vi "Internal Message Loop.vi"(8 "error in (no error)":errorcluster, 11 "WAMP Client in":refnum<class "WAMP Client.lvclass">) -> (0 "error out":errorcluster, 3 "WAMP Client out":refnum<class "WAMP Client.lvclass">)   [LabVIEW 2020, in "wamplv.lvlib" / "WAMP Client.lvclass"]
uses:
  <userlib>/wamplv/WAMP Client/WAMP Client.lvclass
  <userlib>/wamplv/WAMP Client/TypeDef/SUBSCRIBE Requests Map.ctl
  <userlib>/wamplv/WAMP Client/TypeDef/SUBSCRIBE Request Data.ctl
  <userlib>/wamplv/WAMP Client/TypeDef/Subscribe Result.ctl
  <userlib>/wamplv/WAMP Client/TypeDef/Event Payload.ctl
  <userlib>/wamplv/WAMP Client/TypeDef/Subscriptions Map.ctl
  <userlib>/wamplv/WAMP Client/TypeDef/Subscription Details.ctl
  <userlib>/wamplv/WAMP Client/TypeDef/Unsubscribe Requests Map.ctl
  <userlib>/wamplv/WAMP Client/TypeDef/UNSUBSCRIBE Request Data.ctl
  <userlib>/wamplv/WAMP Client/TypeDef/UNSUBSCRIBE Result.ctl
  <userlib>/wamplv/WAMP Client/TypeDef/Message Loop Shift Reg Data.ctl
  <userlib>/wamplv/WAMP Client/TypeDef/REGISTER Request Data.ctl
  <userlib>/wamplv/WAMP Client/TypeDef/REGISTERED or ERROR payload.ctl
  <userlib>/wamplv/WAMP Client/TypeDef/WAMP Error Payload.ctl
  <userlib>/wamplv/WAMP Client/TypeDef/INVOCATION payload.ctl
  <userlib>/wamplv/WAMP Client/TypeDef/Publish Requests Map.ctl
  <userlib>/wamplv/WAMP Client/TypeDef/PUBLISH Request Data.ctl
  <userlib>/wamplv/WAMP Client/TypeDef/PUBLISH Result.ctl
  <userlib>/wamplv/WAMP Client/TypeDef/Endpoint Data.ctl
  <userlib>/wamplv/WAMP Client/TypeDef/CALL Request Map.ctl
  <userlib>/wamplv/WAMP Client/TypeDef/CALL Request Data.ctl
  <userlib>/wamplv/WAMP Client/TypeDef/RESULT Payload.ctl
  <userlib>/wamplv/WAMP Client/WAMP Client.lvclass/WAMP Client.ctl
  <userlib>/wamplv/WAMP Client/TypeDef/WAMP Received Message.ctl
  <userlib>/wamplv/WAMP Message Codes.ctl
  <userlib>/wamplv/WAMP Client/TypeDef/Termination Reason Enum.ctl
  <userlib>/wamplv/WAMP Client/TypeDef/GOODBYE Request Data.ctl
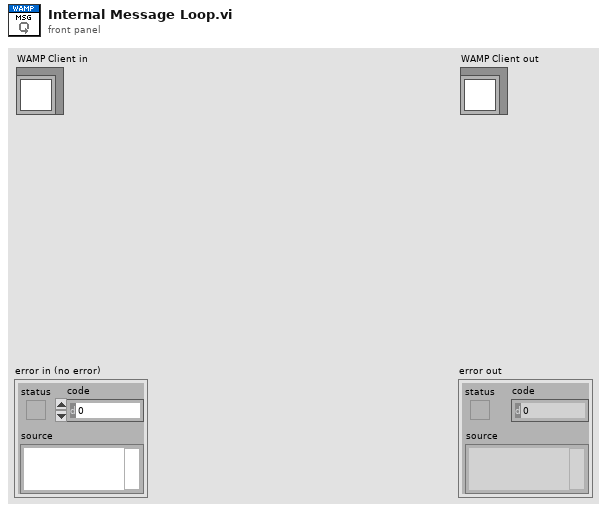
[diagram p1: front panel]
types:
  T1 = typedef "wamplv.lvlib/WAMP Client.lvclass/Message Loop Shift Reg Data.ctl" = cluster{"Register Requests":map{u32, T2}, "Last Request ID":u32, "Publish Requests":T3, "Endpoints Map":map{u32, T5}, "Call Requests":T6}
  T2 = typedef "wamplv.lvlib/WAMP Client.lvclass/REGISTER Request Data.ctl" = cluster{"Procedure URI":string, "Options":string, "REGISTERED or ERROR event":refnum<user-event>, "INVOCATION event":refnum<user-event>}
  T3 = typedef "wamplv.lvlib/WAMP Client.lvclass/Publish Requests Map.ctl" = map{u32, T4}
  T4 = typedef "wamplv.lvlib/WAMP Client.lvclass/PUBLISH Request Data.ctl" = cluster{"Topic URI":string, "Arguments":variant[], "ArgumentsKw":string, "Publish Result Event":refnum<user-event>, "Request Ackoweldegemtn":bool}
  T5 = typedef "wamplv.lvlib/WAMP Client.lvclass/Endpoint Data.ctl" = cluster{"Procedure URI":string, "INVOCATION event":refnum<user-event>}
  T6 = typedef "wamplv.lvlib/WAMP Client.lvclass/CALL Request Map.ctl" = map{u32, T7}
  T7 = typedef "wamplv.lvlib/WAMP Client.lvclass/CALL Request Data.ctl" = cluster{"Topic URI":string, "Arguments":variant[], "ArgumentsKw":string, "Result Received":refnum<user-event>}
  T8 = typedef "wamplv.lvlib/WAMP Client.lvclass/Unsubscribe Requests Map.ctl" = map{u32, T9}
  T9 = typedef "wamplv.lvlib/WAMP Client.lvclass/UNSUBSCRIBE Request Data.ctl" = cluster{"Topic":string, "Unsubscribe Result Received Event":refnum<user-event>}
  T10 = typedef "wamplv.lvlib/WAMP Client.lvclass/Subscriptions Map.ctl" = map{u32, T11}
  T11 = typedef "wamplv.lvlib/WAMP Client.lvclass/Subscription Details.ctl" = cluster{"Subscription ID":u32, "Topic":string, "Publication Received Event":refnum<user-event>}
  T12 = typedef "wamplv.lvlib/WAMP Client.lvclass/SUBSCRIBE Requests Map.ctl" = map{u32, T13}
  T13 = typedef "wamplv.lvlib/WAMP Client.lvclass/SUBSCRIBE Request Data.ctl" = cluster{"Topic":string, "Subscribe Response Received Event":refnum<user-event>}
  T14 = typedef "wamplv.lvlib/WAMP Client.lvclass/Termination Reason Enum.ctl" = enum16{"Goodbye Received", "Abort Received", "Send Goodbye", "Send Abort", "Read Loop Failure", "Write Loop Failure", "Message Loop Failure"}
  T15 = typedef "wamplv.lvlib/WAMP Client.lvclass/WAMP Received Message.ctl" = cluster{"Message JSON":string[], "Message Codes":T16}
  T16 = typedef "wamplv.lvlib/WAMP Client.lvclass/WAMP Message Codes.ctl" = u16
  T17 = typedef "wamplv.lvlib/WAMP Client.lvclass/GOODBYE Request Data.ctl" = cluster{"Error URI":string, "Message":string}
  T18 = typedef "wamplv.lvlib/WAMP Client.lvclass/Internal Message.ctl" = cluster{"Internal Message Type":T19, "Variant":variant}
  T19 = typedef "wamplv.lvlib/WAMP Client.lvclass/Internal Message Type.ctl" = enum16{"Subscribe", "Handle Subscribed", "Handle Event", "Unsubscribe", "Handle Unsubscribed", "Publish", "Handled Published", "Goodbye", "Handle Goodbye", "Call", "Handle Result", "Register", "Handle Registered", "Unregister", "Handle Unregistered", "Handle Invocation", "Yield", "Error"}
  T20 = typedef "wamplv.lvlib/WAMP Client.lvclass/YIELD request data.ctl" = cluster{"Invocation Request ID":u32, "Arguments":variant[], "ArgumentsKw":string, "Options":string}
  T21 = typedef "wamplv.lvlib/WAMP Client.lvclass/Error Request.ctl" = cluster{"WAMP Error":T22, "Message Type":T16, "Request ID":u32}
  T22 = typedef "wamplv.lvlib/WAMP Client.lvclass/WAMP Error Payload.ctl" = cluster{"Details":string, "ArgumentKw Payload":string, "Error?":bool, "Error URI":string, "Arguments Payload":string[]}
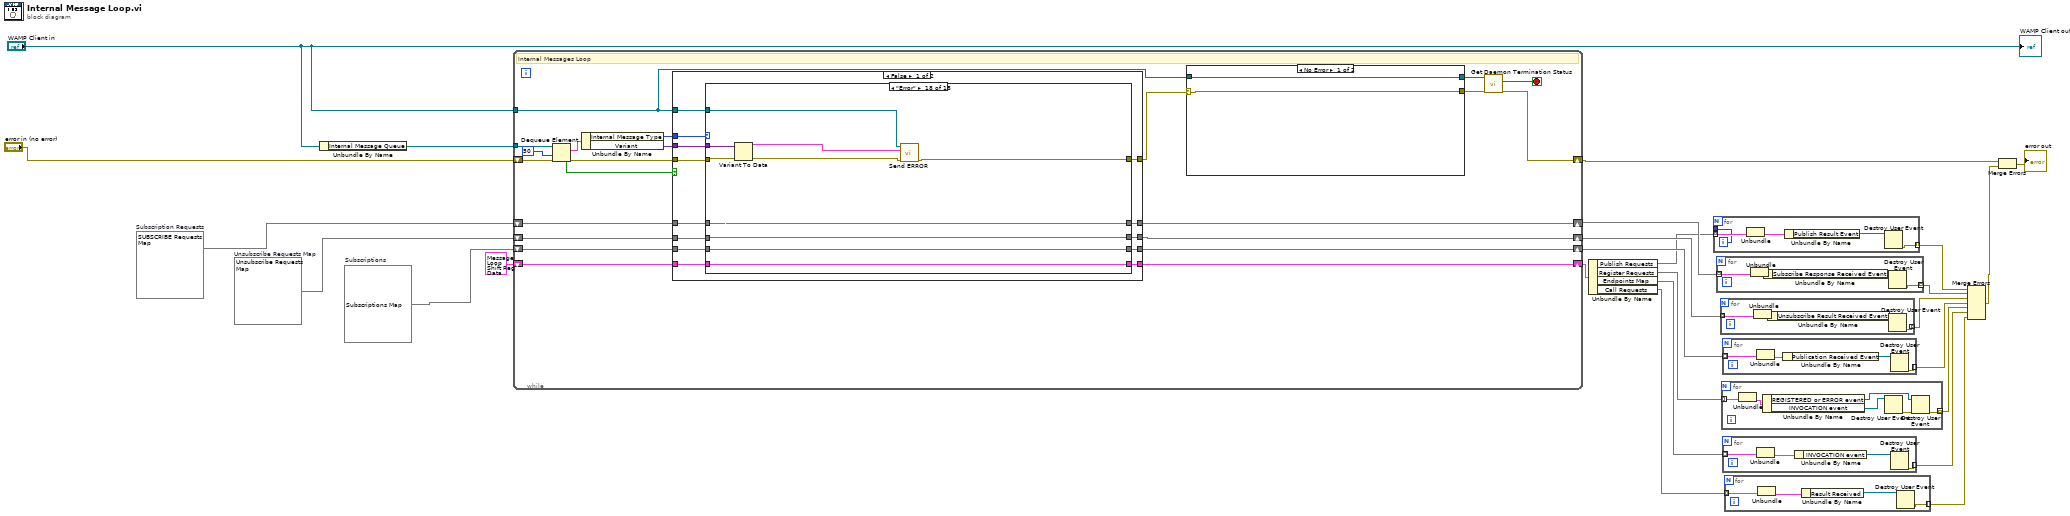
[diagram p0: block diagram]
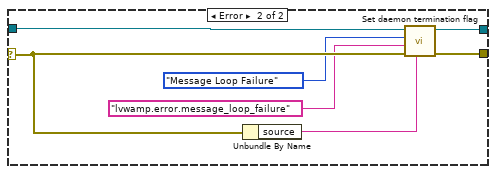
[diagram p2: hidden frame]
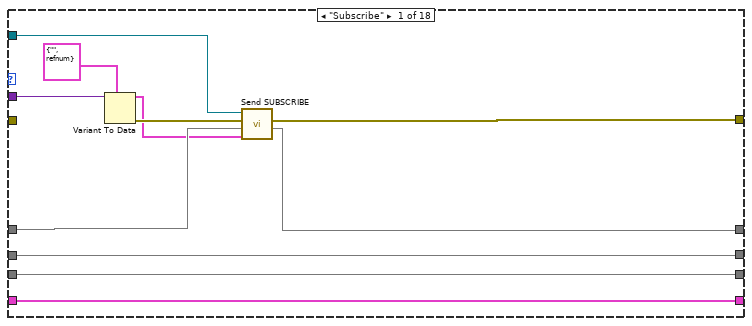
[diagram p3: hidden frame]
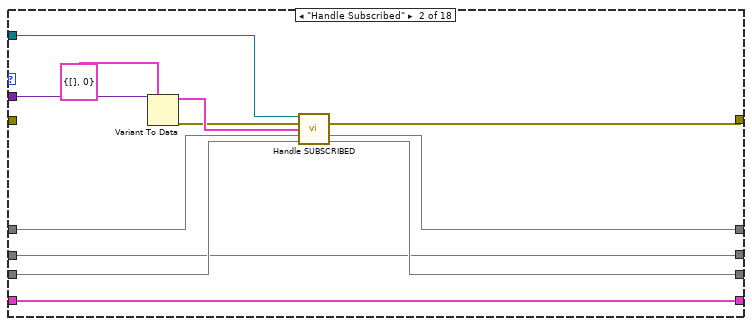
[diagram p4: hidden frame]
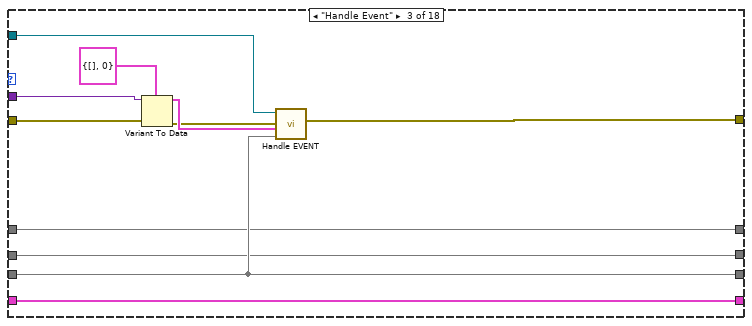
[diagram p5: hidden frame]
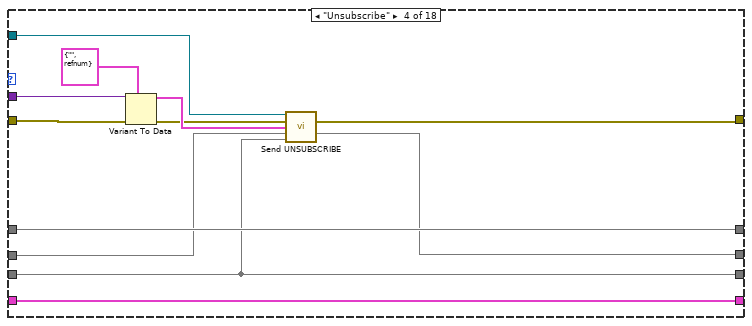
[diagram p6: hidden frame]
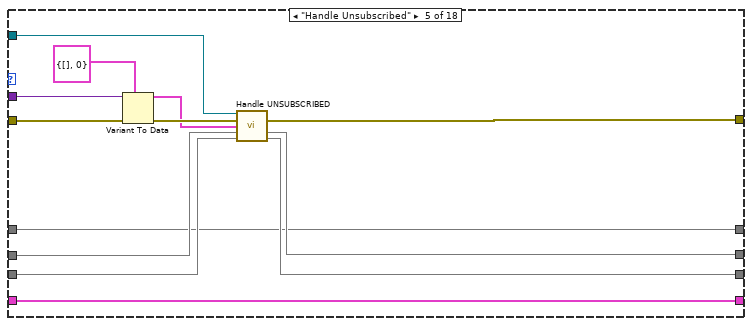
[diagram p7: hidden frame]
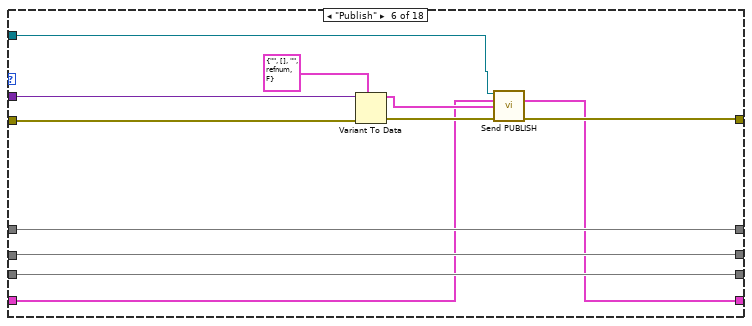
[diagram p8: hidden frame]
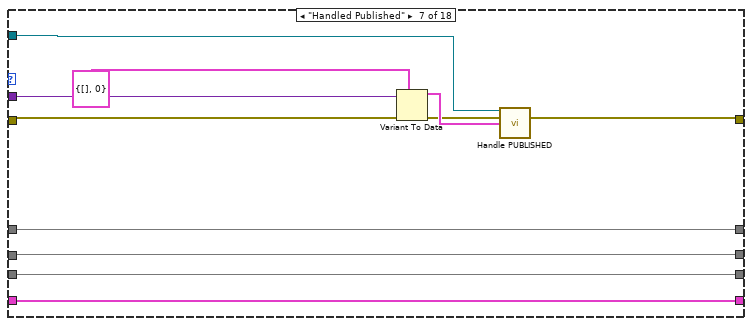
[diagram p9: hidden frame]
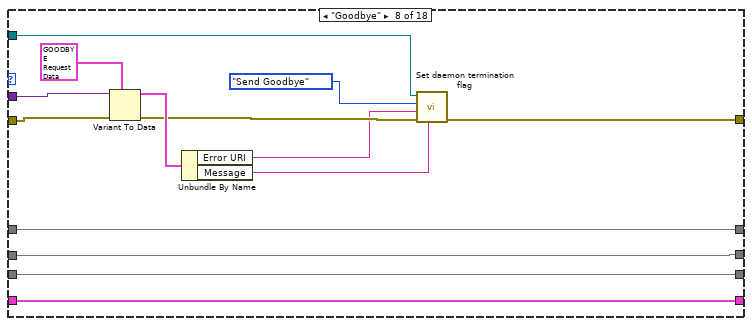
[diagram p10: hidden frame]
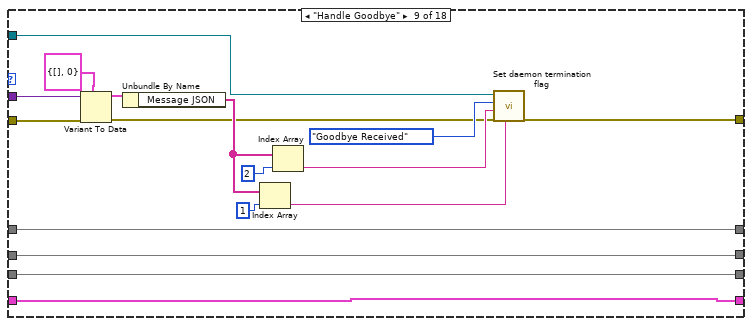
[diagram p11: hidden frame]
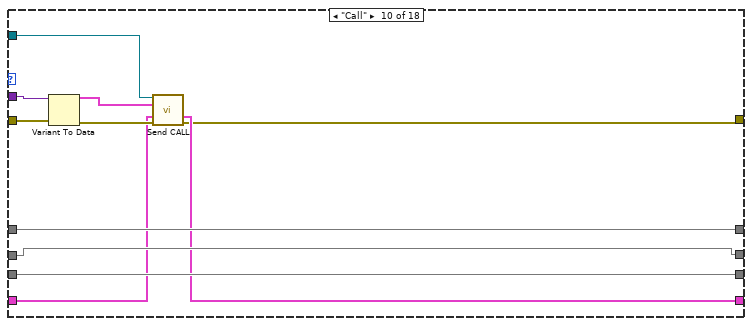
[diagram p12: hidden frame]
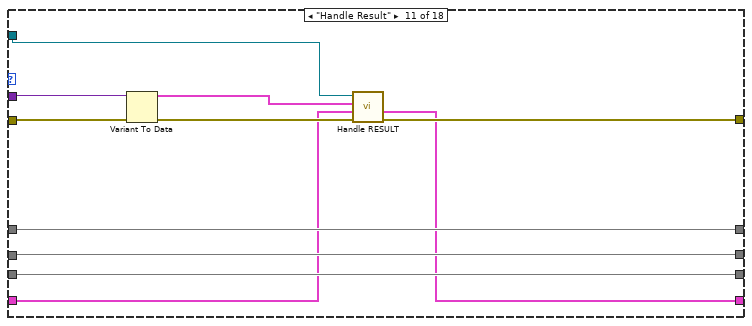
[diagram p13: hidden frame]
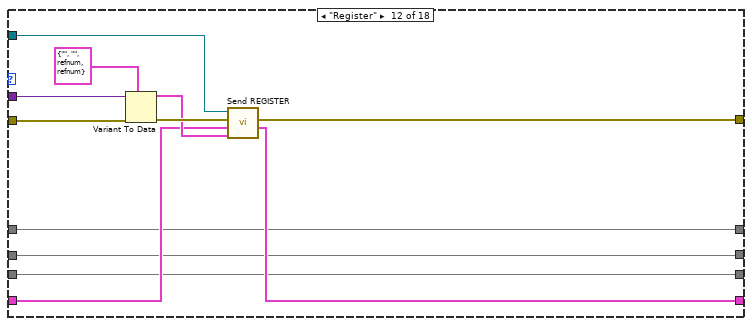
[diagram p14: hidden frame]
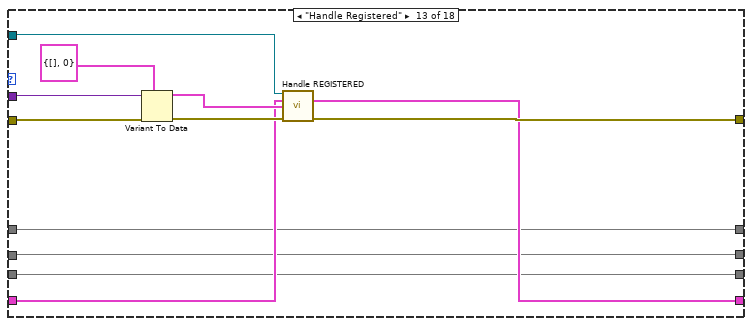
[diagram p15: hidden frame]
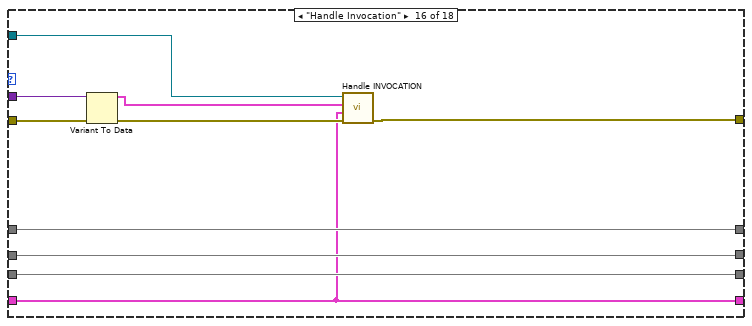
[diagram p18: hidden frame]
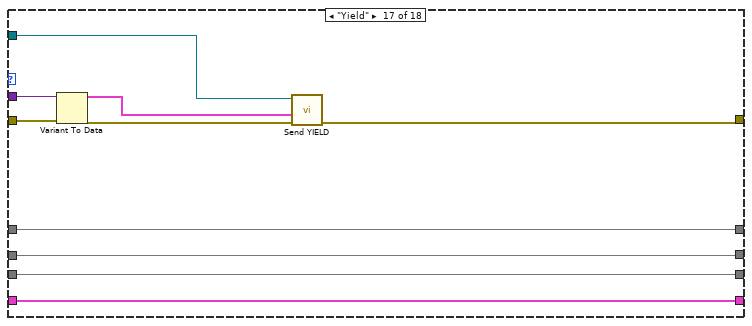
[diagram p19: hidden frame]
diagram:
  w22 = T8 {}  # Unsubscribe Requests Map
  w24 = T10 {}  # Subscriptions
  w25 = T12 {}  # Subscription Requests
  n1 = Unbundle By Name("WAMP Client in") -> ("Internal Message Queue"=w23:refnum<queue>)
  n2 = while {
    tunnel: w23 -> [w46]
    tunnel: "WAMP Client in" -> [w26]
    shift-right: [w41] -> w20
    shift-left: w25 -> [w42]
    shift-right: [w39] -> w18
    shift-left: w24 -> [w40]
    shift-right: [w37] -> w19
    shift-left: w22 -> [w38]
    shift-right: [w28] -> w10
    shift-left: "error in (no error)" -> [w35]
    shift-right: [w31] -> w8
    shift-left: T1 {"Register Requests"={}, "Last Request ID"=0, "Publish Requests"={}, "Endpoints Map"={}, "Call Requests"={}} ("Message Loop Shift Register Data") -> [w32]
    stop <- w27 stop-if-true
    # "Internal Messages Loop"
    n3 = Dequeue Element(queue=w46, timeout in ms (-1)=50, error in (no error)=w35) -> (element=w45:T18, timed out?=w36:bool, error out=w34:errorcluster)  [unwired: 1 out]
    n4 = Unbundle By Name(w45) -> ("Internal Message Type"=w44:T19, "Variant"=w43:variant)
    n5 = case shown="False" w36 {
      tunnel: w44 -> [w69 _]
      tunnel: w43 -> [w68 _]
      tunnel: w26 -> [w67 _]
      tunnel: w42 -> [w66 w273]
      tunnel: [w65 w273] -> w41
      tunnel: w40 -> [w64 w271]
      tunnel: [w63 w271] -> w39
      tunnel: w38 -> [w62 w272]
      tunnel: [w61 w272] -> w37
      tunnel: w34 -> [w60 w270]
      tunnel: [w59 w270] -> w33
      tunnel: w32 -> [w58 w269]
      tunnel: [w57 w269] -> w31
      frame False {
        n6 = case shown="\"Error\"" w69 {
          tunnel: w68 -> [w80 w91 w100 w115 w128 w137 w150 w165 w176 w193 w203 w215 w228 _ _ w244 w254 w264]
          tunnel: w67 -> [w78 w92 w103 w113 w126 w132 w142 w155 w166 w191 w204 w210 w224 _ _ w245 w250 w267]
          tunnel: w66 -> [w76 w87 w101 w114 w119 w140 w148 w161 w182 w188 w199 w207 w219 w233 w238 w248 w258 w262]
          tunnel: [w75 w85 w101 w114 w119 w140 w148 w161 w182 w188 w199 w207 w219 w233 w238 w248 w258 w262] -> w65
          tunnel: w64 -> [w73 w86 w102 w108 w121 w138 w146 w159 w180 w190 w201 w205 w217 w231 w236 w246 w256 w260]
          tunnel: [w73 w84 w102 w108 w120 w138 w146 w159 w180 w190 w201 w205 w217 w231 w236 w246 w256 w260] -> w63
          tunnel: w62 -> [w72 w83 w97 w110 w123 w139 w147 w160 w181 w189 w200 w206 w218 w232 w237 w247 w257 w261]
          tunnel: [w72 w83 w97 w109 w122 w139 w147 w160 w181 w189 w200 w206 w218 w232 w237 w247 w257 w261] -> w61
          tunnel: w60 -> [_ _ w95 w106 w118 w134 w144 w163 w177 w192 w202 w213 w227 w229 w234 w243 w253 w265]
          tunnel: [w71 w82 w96 w105 w117 w130 w143 w157 w178 w183 w197 w209 w222 w229 w234 w241 w249 w268] -> w59
          tunnel: w58 -> [w70 w81 w93 w104 w116 w131 w141 w158 w179 w185 w195 w211 w221 w230 w235 w239 w255 w259]
          tunnel: [w70 w81 w93 w104 w116 w129 w141 w158 w179 w184 w194 w208 w220 w230 w235 w239 w255 w259] -> w57
          frame "Subscribe" {
            n7 = Variant To Data(type=T13 {"Topic"="", "Subscribe Response Received Event"=refnum} ("Cluster"), Variant=w80) -> (data=w74:T13, error out=w77:errorcluster)  [unwired: 1 in]
            n8 = call-dynamic "Send SUBSCRIBE.vi"("Subscription Request"=w74, "Subscription Requests Map"=w76, "error in (no error)"=w77, "WAMP Client in"=w78) -> ("Subscription Requests List 2"=w75:map{u32, T13}, "error out"=w71:errorcluster)  [unwired: 5 in, 1 out]
          }
          frame "Handle Subscribed" {
            n9 = Variant To Data(type=T15 {"Message JSON"=[], "Message Codes"=0} ("Cluster"), Variant=w91) -> (data=w89:T15, error out=w88:errorcluster)  [unwired: 1 in]
            n10 = call-dynamic "Handle SUBSCRIBED.vi"("reference"=w92, "error in (no error)"=w88, "WAMP Message"=w89, "Subscription Requests In"=w87, "Subscriptions In"=w86) -> ("error out"=w82:errorcluster, "Subscription Requests Out"=w85:map{u32, T13}, "Subscriptions Map Out"=w84:map{u32, T11})  [unwired: 7 in, 1 out]
          }
          frame "Handle Event" {
            n11 = Variant To Data(error in=w95, type=T15 {"Message JSON"=[], "Message Codes"=0} ("Cluster"), Variant=w100) -> (data=w99:T15, error out=w94:errorcluster)
            n12 = call-dynamic "Handle EVENT.vi"("Subscriptions"=w102, "Cluster"=w99, "error in (no error)"=w94, "reference"=w103) -> ("error out"=w96:errorcluster)  [unwired: 6 in, 1 out]
          }
          frame "Unsubscribe" {
            n13 = Variant To Data(error in=w106, type=T9 {"Topic"="", "Unsubscribe Result Received Event"=refnum} ("Cluster"), Variant=w115) -> (data=w112:T9, error out=w107:errorcluster)
            n14 = call-dynamic "Send UNSUBSCRIBE.vi"("WAMP Client in"=w113, "error in (no error)"=w107, "Unsubscribe Request Data"=w112, "Unsubscribe Requests Map (in)"=w110, "Subscriptions"=w108) -> ("error out"=w105:errorcluster, "Unsubscribe Requests Map (out)"=w109:T8)  [unwired: 8 in, 1 out]
          }
          frame "Handle Unsubscribed" {
            n15 = Variant To Data(error in=w118, type=T15 {"Message JSON"=[], "Message Codes"=0} ("Cluster"), Variant=w128) -> (data=w124:T15, error out=w125:errorcluster)
            n16 = call-dynamic "Handle UNSUBSCRIBED.vi"("reference"=w126, "error in (no error)"=w125, "WAMP Message"=w124, "Unsubscribe Reqeusts (in)"=w123, "Subscriptions In"=w121) -> ("error out"=w117:errorcluster, "Unsubscribe Reqeusts (out)"=w122:T8, "Subscriptions Map Out"=w120:map{u32, T11})  [unwired: 7 in, 1 out]
          }
          frame "Publish" {
            n17 = Variant To Data(error in=w134, type=T4 {"Topic URI"="", "Arguments"=[], "ArgumentsKw"="", "Publish Result Event"=refnum, "Request Ackoweldegemtn"=FALSE} ("Cluster"), Variant=w137) -> (data=w135:T4, error out=w133:errorcluster)
            n18 = call-dynamic "Send PUBLISH.vi"("WAMP Client in"=w132, "Message Loop Shift Register Data (In)"=w131, "Publish Request Data"=w135, "error in (no error)"=w133) -> ("Message Loop Shift Register Data (Out)"=w129:T1, "error out"=w130:errorcluster)  [unwired: 9 in, 1 out]
          }
          frame "Handled Published" {
            n19 = Variant To Data(error in=w144, type=T15 {"Message JSON"=[], "Message Codes"=0} ("Cluster"), Variant=w150) -> (data=w149:T15, error out=w145:errorcluster)
            n20 = call-dynamic "Handle PUBLISHED.vi"("reference"=w142, "error in (no error)"=w145, "WAMP Message"=w149) -> ("error out"=w143:errorcluster)  [unwired: 10 in, 2 out]
          }
          frame "Goodbye" {
            n21 = Variant To Data(error in=w163, type=T17 {"Error URI"="wamp.error.protocol_violation", "Message"="wamp.close.shut_down"} ("Goodbye Request"), Variant=w165) -> (data=w162:T17, error out=w156:errorcluster)
            n22 = Unbundle By Name(w162) -> ("Error URI"=w153:string, "Message"=w152:string)
            n23 = call <userlib>:"Set daemon termination flag.vi"("Message"=w152, "error in (no error)"=w156, "Reason URI"=w153, "Reason"=Termination_Reason_Enum."Send Goodbye" ("Termination Reason"), "WAMP Client (in)"=w155) -> ("error out"=w157:errorcluster)  [unwired: 5 in, 1 out]
          }
          frame "Handle Goodbye" {
            n24 = Variant To Data(error in=w177, type=T15 {"Message JSON"=[], "Message Codes"=0} ("Cluster"), Variant=w176) -> (data=w174:T15, error out=w167:errorcluster)
            n25 = Unbundle By Name(w174) -> ("Message JSON"=w171:string[])
            n26 = Index Array(array=w171, index=1) -> (element=w168:string)
            n27 = Index Array(array=w171, index=2) -> (element=w169:string)
            n28 = call <userlib>:"Set daemon termination flag.vi"("Message"=w168, "error in (no error)"=w167, "Reason URI"=w169, "Reason"=Termination_Reason_Enum."Goodbye Received" ("Termination Reason"), "WAMP Client (in)"=w166) -> ("error out"=w178:errorcluster)  [unwired: 5 in, 1 out]
          }
          frame "Call" {
            n29 = Variant To Data(error in=w192, Variant=w193) -> (data=w186:T7, error out=w187:errorcluster)  [unwired: 1 in]
            n30 = call-dynamic "Send CALL.vi"("WAMP Client in"=w191, "Call Request"=w186, "Message Loop Shift Register Data"=w185, "error in (no error)"=w187) -> ("Message Loop Shift Register Data (out)"=w184:T1, "error out"=w183:errorcluster)  [unwired: 9 in, 1 out]
          }
          frame "Handle Result" {
            n31 = Variant To Data(error in=w202, Variant=w203) -> (data=w198:T15, error out=w196:errorcluster)  [unwired: 1 in]
            n32 = call-dynamic "Handle RESULT.vi"("error in (no error)"=w196, "Message Loop Shift Register Data"=w195, "WAMP Message"=w198, "reference"=w204) -> ("error out"=w197:errorcluster, "Message Loop Shift Register Data (out)"=w194:T1)  [unwired: 5 in, 1 out]
          }
          frame "Register" {
            n33 = Variant To Data(error in=w213, type=T2 {"Procedure URI"="", "Options"="", "REGISTERED or ERROR event"=refnum, "INVOCATION event"=refnum} ("REGISTER request data"), Variant=w215) -> (data=w212:T2, error out=w214:errorcluster)
            n34 = call-dynamic "Send REGISTER.vi"("REGISTER request data"=w212, "Message Loop Shift Register Data"=w211, "error in (no error)"=w214, "WAMP Client in"=w210) -> ("Message Loop Shift Register Data"=w208:T1, "error out"=w209:errorcluster)  [unwired: 5 in, 1 out]
          }
          frame "Handle Registered" {
            n35 = Variant To Data(error in=w227, type=T15 {"Message JSON"=[], "Message Codes"=0} ("Cluster"), Variant=w228) -> (data=w226:T15, error out=w223:errorcluster)
            n36 = call-dynamic "Handle REGISTERED.vi"("reference"=w224, "Message Loop Shift Register Data"=w221, "WAMP Message"=w226, "error in (no error)"=w223) -> ("output cluster"=w220:T1, "error out"=w222:errorcluster)  [unwired: 9 in, 1 out]
          }
          frame "Unregister" {
          }
          frame "Handle Unregistered" {
          }
          frame "Handle Invocation" {
            n37 = Variant To Data(error in=w243, Variant=w244) -> (data=w240:T15, error out=w242:errorcluster)  [unwired: 1 in]
            n38 = call-dynamic "Handle INVOCATION.vi"("error in (no error)"=w242, "Message Loop Shift Register Data"=w239, "Cluster"=w240, "reference"=w245) -> ("error out"=w241:errorcluster)  [unwired: 6 in, 1 out]
          }
          frame "Yield" {
            n39 = Variant To Data(error in=w253, Variant=w254) -> (data=w252:T20, error out=w251:errorcluster)  [unwired: 1 in]
            n40 = call-dynamic "Send YIELD.vi"("error in (no error)"=w251, "Yield request"=w252, "WAMP Client in"=w250) -> ("error out"=w249:errorcluster)  [unwired: 7 in, 1 out]
          }
          frame "Error" {
            n41 = Variant To Data(error in=w265, Variant=w264) -> (data=w263:T21, error out=w266:errorcluster)  [unwired: 1 in]
            n42 = call-dynamic "Send ERROR.vi"("error in (no error)"=w266, "Error Request"=w263, "WAMP Client in"=w267) -> ("error out"=w268:errorcluster)  [unwired: 7 in, 1 out]
          }
        }
      }
      frame True {
        # "Time out, no internal messages"
      }
    }
    n43 = case shown="No Error" w33 {
      selector: w33 -> [w49 w55]
      tunnel: [w49 w56] -> w30
      tunnel: [w48 w54] -> w29
      tunnel: w26 -> [w48 w53]
      frame No Error {
      }
      frame Error {
        n44 = Unbundle By Name(w55) -> ("source"=w50:string)
        n45 = call <userlib>:"Set daemon termination flag.vi"("Message"=w50, "error in (no error)"=w55, "Reason URI"="lvwamp.error.message_loop_failure" ("Error URI"), "Reason"=Termination_Reason_Enum."Message Loop Failure" ("Termination Reason"), "WAMP Client (in)"=w53) -> ("error out"=w56:errorcluster, "WAMP Client (out)"=w54:refnum<class "WAMP Client.lvclass">)  [unwired: 5 in]
      }
    }
    n46 = call <userlib>:"Get Daemon Termination Status.vi"("error in (no error)"=w30, "WAMP Client in"=w29) -> ("error out"=w28:errorcluster, "Terminate?"=w27:bool)  [unwired: 6 in, 2 out]
  }
  n47 = Unbundle By Name(w8) -> ("Publish Requests"=w7:T3, "Register Requests"=w6:map{u32, T2}, "Endpoints Map"=w4:map{u32, T5}, "Call Requests"=w2:T6)
  n48 = for {
    tunnel: w7 -> [w278] mode=indexing
    tunnel: [w276] -> w13 mode=indexing
    tunnel: [w275] -> _
    i -> [w275]
    n49 = Unbundle(w278) -> (w277:T4)  [unwired: 1 out]
    n50 = Unbundle By Name(w277) -> ("Publish Result Event"=w274:refnum<user-event>)
    n51 = Destroy User Event(user event=w274) -> (error out=w276:errorcluster)  [unwired: 1 in]
  }
  n52 = for {
    tunnel: w20 -> [w282] mode=indexing
    tunnel: [w279] -> w14 mode=indexing
    n53 = Unbundle(w282) -> (w281:T13)  [unwired: 1 out]
    n54 = Unbundle By Name(w281) -> ("Subscribe Response Received Event"=w280:refnum<user-event>)
    n55 = Destroy User Event(user event=w280) -> (error out=w279:errorcluster)  [unwired: 1 in]
  }
  n56 = for {
    tunnel: w19 -> [w286] mode=indexing
    tunnel: [w283] -> w15 mode=indexing
    n57 = Unbundle(w286) -> (w285:T9)  [unwired: 1 out]
    n58 = Unbundle By Name(w285) -> ("Unsubscribe Result Received Event"=w284:refnum<user-event>)
    n59 = Destroy User Event(user event=w284) -> (error out=w283:errorcluster)  [unwired: 1 in]
  }
  n60 = for {
    tunnel: w6 -> [w292] mode=indexing
    tunnel: [w287] -> w5 mode=indexing
    n61 = Unbundle(w292) -> (w291:T2)  [unwired: 1 out]
    n62 = Unbundle By Name(w291) -> ("REGISTERED or ERROR event"=w290:refnum<user-event>, "INVOCATION event"=w289:refnum<user-event>)
    n63 = Destroy User Event(user event=w289) -> (error out=w288:errorcluster)  [unwired: 1 in]
    n64 = Destroy User Event(user event=w290, error in=w288) -> (error out=w287:errorcluster)
  }
  n65 = for {
    tunnel: w18 -> [w296] mode=indexing
    tunnel: [w293] -> w16 mode=indexing
    n66 = Unbundle(w296) -> (w295:T11)  [unwired: 1 out]
    n67 = Unbundle By Name(w295) -> ("Publication Received Event"=w294:refnum<user-event>)
    n68 = Destroy User Event(user event=w294) -> (error out=w293:errorcluster)  [unwired: 1 in]
  }
  n69 = for {
    tunnel: w4 -> [w300] mode=indexing
    tunnel: [w297] -> w3 mode=indexing
    n70 = Unbundle(w300) -> ("Endpoint Data"=w299:T5)  [unwired: 1 out]
    n71 = Unbundle By Name(w299) -> ("INVOCATION event"=w298:refnum<user-event>)
    n72 = Destroy User Event(user event=w298) -> (error out=w297:errorcluster)  [unwired: 1 in]
  }
  n73 = for {
    tunnel: w2 -> [w304] mode=indexing
    tunnel: [w302] -> w1 mode=indexing
    n74 = Unbundle(w304) -> (w303:T7)  [unwired: 1 out]
    n75 = Unbundle By Name(w303) -> ("Result Received"=w301:refnum<user-event>)
    n76 = Destroy User Event(user event=w301) -> (error out=w302:errorcluster)  [unwired: 1 in]
  }
  n77 = Merge Errors(w13, w14, w15, w16, w5, w3, w1) -> (w11:errorcluster)
  n78 = Merge Errors(w10, w11) -> (→"error out":errorcluster)
  "WAMP Client out" <- "WAMP Client in"
